vi "Splash UI.vi"(11 "Basic Splash in":refnum<class "Basic Splash.lvclass">) -> ()   [LabVIEW 2020, in "Volatus.lvlib" / "Basic Splash.lvclass"]
uses:
  Basic Splash.lvclass
  Basic Splash.lvclass/Basic Splash.ctl
panel:
  out "Status":string
  # "VOLATUS"
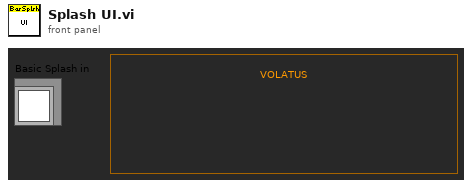
[diagram p1: front panel]
types:
  T1 = enum32{"Invalid", "Standard", "Closed", "Hidden", "Minimized", "Maximized"}
  T2 = typedef "Volatus.lvlib/Basic Splash.lvclass/Event Type.ctl" = enum16{"Show", "Hide", "Update", "Close"}
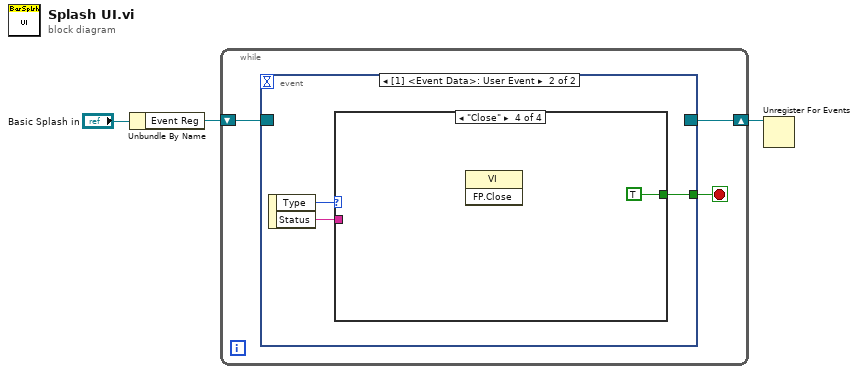
[diagram p0: block diagram]
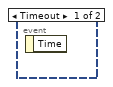
[diagram p2: hidden frame]
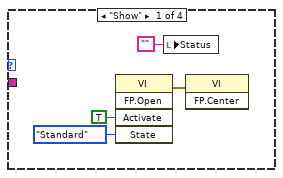
[diagram p3: hidden frame]
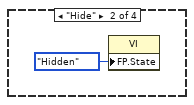
[diagram p4: hidden frame]
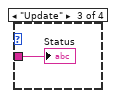
[diagram p5: hidden frame]
diagram:
  n1 = Unbundle By Name("Basic Splash in") -> ("Event Reg"=w2:refnum<event-registration>)
  n2 = while {
    shift-right: [w5] -> w1
    shift-left: w2 -> [w6]
    stop <- w4 stop-if-true
    n3 = event shown="[1] <Event Data>: User Event" {
      selector: w6 -> [_ _]
      dyn-events: [_ _] -> w5
      timeout: _ -> [_ _]
      tunnel: [_ w7] -> w4
      event Timeout {
        n4 = event-data() -> ()  [unwired: 1 in, 1 out]
      }
      event User Event {
        n5 = event-data() -> ("Type"=w9:T2, "Status"=w8:string)  [unwired: 1 in]
        n6 = case shown="\"Close\"" w9 {
          tunnel: w8 -> [_ _ w15 _]
          tunnel: [_ _ _ TRUE] -> w7
          frame "Show" {
            n7 = invoke class="VI" method="FP.Open"("Activate"=TRUE ("Activate?"), "State"=T1."Standard") -> (error out=w10:errorcluster)  [unwired: 3 in, 4 out]
            n8 = local write "Status"("") -> ()
            n9 = invoke class="VI" method="FP.Center"(error in=w10) -> ()  [unwired: 2 in, 3 out]
          }
          frame "Hide" {
            n10 = property class="VI"("FP.State"=T1."Hidden" ("Front Panel Window:State")) -> ()  [unwired: 2 in, 2 out]
          }
          frame "Update" {
            "Status" <- w15
          }
          frame "Close" {
            n11 = invoke class="VI" method="FP.Close"() -> ()  [unwired: 3 in, 3 out]
          }
        }
      }
    }
  }
  n12 = Unregister For Events(event registration refnum=w1) -> ()  [unwired: 1 in, 1 out]
